vi "Swerve Wheel.vi"(7 "Wheel":T1(ring), 10 "Inputs":dbl[](array[numeric])) -> (1 "Speed":dbl, 2 "Motor Output":dbl)   [LabVIEW 2017]
uses:
  <vilib>/Rock Robotics/WPI/ThirdParty/Phoenix-LabVIEW/Motor Controller/Controls/CTRE_Phoenix_MotorControl_ControlMode.ctl
  <vilib>/Rock Robotics/Network Tables/NT Read Number.vi
  <vilib>/Rock Robotics/Network Tables/NT Write Number.vi
  <vilib>/Rock Robotics/Network Tables/NT Read Numeric Array.vi
  <vilib>/addons/control/pid/pid.llb/PID (DBL).vi
  <vilib>/addons/control/pid/NI_PID_pid.lvlib
panel:
  out "PID Values":cluster{"P":dbl, "I":dbl, "D":dbl}
  # "Swerve Wheel Control\nFRC Team 34"
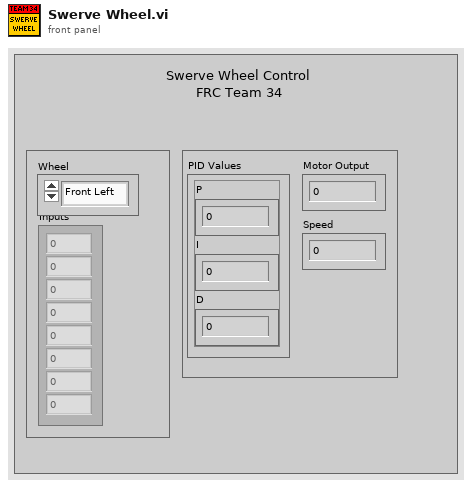
[diagram p1: front panel]
types:
  T1 = enum16{"Front Left", "Front Right", "Back Left", "Back Right"}
  T2 = enum16{"Z Axis", "Y", "X", "Rot. Point X", "Rot. Point Y", "Width/2", "Max", "Length/2"}
  T3 = typedef "CTRE_Phoenix_MotorControl_ControlMode.ctl" = u16
  T4 = enum16{"Z", "Y", "X", "Rot. Point X", "Rot. Point Y", "Width/2", "Max", "Length/2"}
  T5 = typedef "WPI_MotorControlDeviceRef.ctl" = cluster{"DeviceStatus":errorcluster, "Type":T6, "PWM":cluster{"PWM Channel":T7, "DeadBand":T8}, "CAN":cluster{"Device Number":u8, "SetOutput VI Ref":variant, "GetOutput VI Ref":variant, "Enable VI Ref":variant, "Disable VI Ref":variant, "Data":variant}, "Invert":bool, "DIO PWM":cluster{"PWM \"Enable\" Channel":T7, "DIOChannel":T9, "PWM Rate":dbl}}
  T6 = typedef "WPI_MotorControlType.ctl" = enum16{"PWM", "CAN", "DIO PWM"}
  T7 = typedef "FPGA_DIOPWMChannel.ctl" = enum8{"PWM 0", "PWM 1", "PWM 2", "PWM 3", "PWM 4", "PWM 5", "PWM 6", "PWM 7", "PWM 8", "PWM 9", "PWM MXP 0", "PWM MXP 1", "PWM MXP 2", "PWM MXP 3", "PWM MXP 4", "PWM MXP 5", "PWM MXP 6", "PWM MXP 7", "PWM MXP 8", "PWM MXP 9", "Invalid"}
  T8 = typedef "WPI_PWMDeadband.ctl" = cluster{"Name":string, "maxPositivePwm":i32, "minPositivePwm":i32, "centerPwm":i32, "maxNegativePwm":i32, "minNegativePwm":i32, "angularRange":u16}
  T9 = typedef "FPGA_DIOChannel.ctl" = enum8{"DIO 0", "DIO 1", "DIO 2", "DIO 3", "DIO 4", "DIO 5", "DIO 6", "DIO 7", "DIO 8", "DIO 9", "DIO MXP 0", "DIO MXP 1", "DIO MXP 2", "DIO MXP 3", "DIO MXP 4", "DIO MXP 5", "DIO MXP 6", "DIO MXP 7", "DIO MXP 8", "DIO MXP 9", "DIO MXP 10", "DIO MXP 11", "DIO MXP 12", "DIO MXP 13", "DIO MXP 14", "DIO MXP 15", "SPI Port CS1", "SPI Port CS2", "SPI Port CS3", "SPI Port MISO", "SPI Port MOSI", "Invalid"}
  T10 = typedef "WPI_EncoderDevRef.ctl" = cluster{"DevStatus":errorcluster, "EncoderIndex":T11, "CounterIndex":T12, "DistancePerCount":dbl, "Decoding Type":T13}
  T11 = typedef "FPGA_EncoderIdx.ctl" = enum8{"Enc 0", "Enc 1", "Enc 2", "Enc 3", "Enc 4", "Enc 5", "Enc 6", "Enc 7", "Invalid"}
  T12 = typedef "FPGA_CounterCtrSystemIndex.ctl" = enum8{"Ctr 0", "Ctr 1", "Ctr 2", "Ctr 3", "Ctr 4", "Ctr 5", "Ctr 6", "Ctr 7", "Invalid"}
  T13 = typedef "WPI_EncoderType.ctl" = enum16{"1x", "2x", "4x"}
  T14 = cluster{"Numeric":dbl, "Numeric":dbl, "Numeric":dbl}
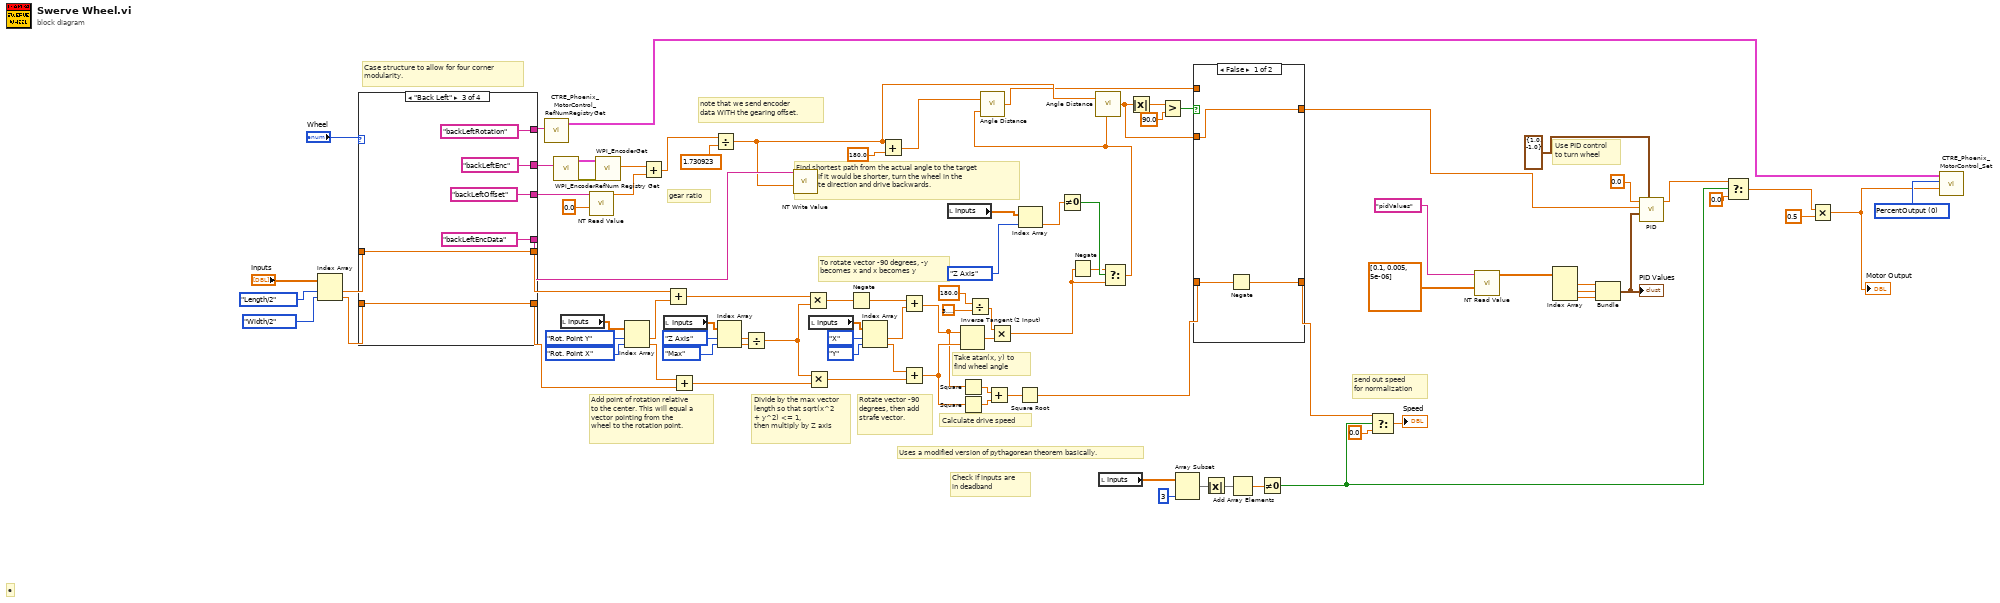
[diagram p0: block diagram]
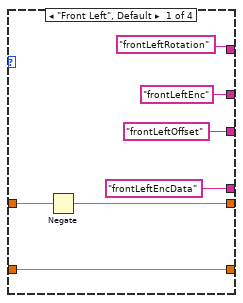
[diagram p3: hidden frame]
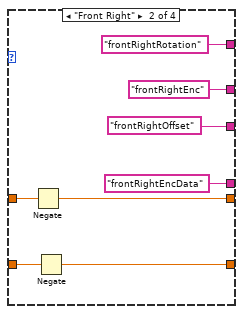
[diagram p4: hidden frame]
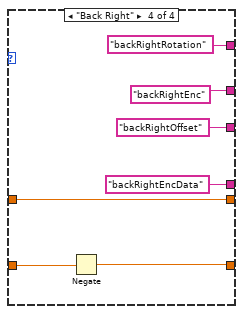
[diagram p5: hidden frame]
diagram:
  w31 = T3 0 items=["PercentOutput"=0, "Position"=1, "Velocity"=2, "Current"=3, "Follower"=5, "MotionProfile"=6, "MotionMagic"=7, "MotionMagicArc"=8, "MotionProfileArc"=10, "Disabled"=15] ("Control Mode")
  # "gear ratio"
  # "Uses a modified version of pythagorean theorem basically."
  # "e"
  # "note that we send encoder \ndata WITH the gearing offset."
  # "Case structure to allow for four corner\nmodularity."
  # "To rotate vector -90 degrees, -y becomes x and x becomes y"
  # "send out speed\nfor normalization"
  # "Use PID control\nto turn wheel"
  # "Find shortest path from the actual angle to the target angle. If it would be shorter, turn the wheel in the opposite direction and drive backwards."
  # "Divide by the max vector length so that sqrt(x^2 + y^2) <= 1,\nthen multiply by Z axis"
  # "Add point of rotation relative to the center. This will equal a vector pointing from the\nwheel to the rotation point."
  # "Check if inputs are\nin deadband"
  # "Take atan(x, y) to find wheel angle"
  # "Calculate drive speed"
  # "Rotate vector -90 degrees, then add strafe vector."
  n1 = Index Array(array="Inputs", index #1=T4."Length/2", index #2=T4."Width/2") -> (element #1=w87:dbl, element #2=w86:dbl)
  n2 = case shown="\"Back Left\"" "Wheel" {
    tunnel: w87 -> [w98 w106 w112 w119]
    tunnel: w86 -> [w96 w104 w111 w118]
    tunnel: [w97 w105 w112 w119] -> w56
    tunnel: [w96 w103 w111 w117] -> w55
    tunnel: ["frontLeftRotation" "frontRightRotation" "backLeftRotation" "backRightRotation"] -> w33
    tunnel: ["frontLeftEnc" ("refnum name") "frontRightEnc" ("refnum name") "backLeftEnc" ("refnum name") "backRightEnc" ("refnum name")] -> w68
    tunnel: ["frontLeftOffset" ("Name") "frontRightOffset" ("Name") "backLeftOffset" ("Name") "backRightOffset" ("Name")] -> w64
    tunnel: ["frontLeftEncData" ("Name") "frontRightEncData" ("Name") "backLeftEncData" ("Name") "backRightEncData" ("Name")] -> w36
    frame "Front Left", Default {
      n3 = Negate(x=w98) -> (-x=w97:dbl)
    }
    frame "Front Right" {
      n4 = Negate(x=w106) -> (-x=w105:dbl)
      n5 = Negate(x=w104) -> (-x=w103:dbl)
    }
    frame "Back Left" {
    }
    frame "Back Right" {
      n6 = Negate(x=w118) -> (-x=w117:dbl)
    }
  }
  n7 = call <vilib>:"CTRE_Phoenix_MotorControl_RefNumRegistryGet.vi"("refnum name"=w33) -> ("PhoenixMotorControlDevRef"=w32:T5)  [unwired: 9 in, 1 out]
  n8 = call <vilib>:"WPI_EncoderRefNum Registry Get.vi"("refnum name"=w68) -> ("error out"=w67:errorcluster, "EncoderDevRef"=w66:T10)  [unwired: 9 in]
  n9 = local read "Inputs"() -> (w61:dbl[])
  n10 = call-poly <vilib>:"NT Read Value.vi"("Default Value"=0.0, "Name"=w64) -> ("Numeric"=w59:dbl)  [unwired: 8 in, 1 out]
  n11 = call <vilib>:"WPI_EncoderGet.vi"("error in (no error)"=w67, "EncoderDevRef"=w66) -> ("Distance"=w60:dbl)  [unwired: 4 in, 5 out]
  n12 = Index Array(array=w61, index #1=T4."Rot. Point Y", index #2=T4."Rot. Point X") -> (element #1=w57:dbl, element #2=w58:dbl)
  n13 = Add(x=w60, y=w59) -> (x+y=w35:dbl)
  n14 = local read "Inputs"() -> (w69:dbl[])
  n15 = Add(x=w56, y=w57) -> (x+y=w54:dbl)
  n16 = Add(x=w58, y=w55) -> (x+y=w78:dbl)
  n17 = Divide(x=w35, y=1.730923) -> (x/y=w24:dbl)
  n18 = Index Array(array=w69, index #1=T2."Z Axis", index #2=T4."Max") -> (element #1=w38:dbl, element #2=w37:dbl)
  n19 = Divide(x=w38, y=w37) -> (x/y=w15:dbl)
  n20 = call-poly <vilib>:"NT Write Value.vi"("Numeric"=w24, "Name"=w36) -> ()  [unwired: 9 in, 1 out]
  n21 = Multiply(x=w54, y=w15) -> (x*y=w71:dbl)
  n22 = Multiply(x=w15, y=w78) -> (x*y=w74:dbl)
  n23 = local read "Inputs"() -> (w41:dbl[])
  n24 = Negate(x=w71) -> (-x=w70:dbl)
  n25 = Index Array(array=w41, index #1=T4."X", index #2=T4."Y") -> (element #1=w40:dbl, element #2=w39:dbl)
  n26 = Add(x=w24, y=180.0) -> (x+y=w23:dbl)
  n27 = Add(x=w70, y=w40) -> (x+y=w72:dbl)
  n28 = Add(x=w39, y=w74) -> (x+y=w73:dbl)
  n29 = local read "Inputs"() -> (w13:dbl[])
  n30 = Inverse Tangent (2 Input)(1:w73, 2:w72) -> (0:w85:dbl)
  n31 = Square(x=w72) -> (x^2=w75:dbl)
  n32 = Square(x=w73) -> (x^2=w84:dbl)
  n33 = Divide(x=180.0 ("y"), y=3.141592653589793) -> (x/y=w82:dbl)
  n34 = Add(x=w75, y=w84) -> (x+y=w83:dbl)
  n35 = Multiply(x=w82, y=w85) -> (x*y=w8:dbl)
  n36 = Square Root(x=w83) -> (sqrt(x)=w21:dbl)
  n37 = Index Array(array=w13, index=T2."Z Axis") -> (element=w11:dbl)
  n38 = Not Equal To 0?(x=w11) -> (x != 0?=w10:bool)
  n39 = Negate(x=w8) -> (-x=w9:dbl)
  n40 = local read "Inputs"() -> (w49:dbl[])
  n41 = Select(t=w9, s=w10, f=w8) -> (s? t:f=w14:dbl)
  n42 = call "Angle Distance.vi"("Target Angle"=w14, "Current Angle"=w23) -> ("Distance"=w22:dbl)
  n43 = call "Angle Distance.vi"("Target Angle"=w14, "Current Angle"=w24) -> ("Distance"=w18:dbl)
  n44 = Absolute Value(x=w18) -> (abs(x)=w17:dbl)
  n45 = Greater?(x=w17, y=90.0) -> (0:w19:bool)
  n46 = Array Subset(array=w49, length=3) -> (w51:dbl[])  [unwired: 1 in]
  n47 = case shown="False" w19 {
    tunnel: w21 -> [w121 w123]
    tunnel: w18 -> [w122 _]
    tunnel: w22 -> [_ w124]
    tunnel: [w120 w123] -> w20
    tunnel: [w122 w124] -> w1
    frame False {
      n48 = Negate(x=w121) -> (-x=w120:dbl)
    }
    frame True {
    }
  }
  n49 = Absolute Value(x=w51) -> (abs(x)=w50:dbl[])
  n50 = Add Array Elements(numeric array=w50) -> (sum=w52:dbl)
  n51 = Not Equal To 0?(x=w52) -> (x != 0?=w42:bool)
  n52 = Select(t=w20, s=w42, f=0.0) -> (s? t:f=→"Speed":dbl)
  n53 = call-poly <vilib>:"NT Read Value.vi"("Default Value"=dbl[] [0.1, 0.005, 5e-06], "Name"="pidValues") -> ("Numeric Array"=w6:dbl[])  [unwired: 8 in, 1 out]
  n54 = Index Array(array=w6) -> (element #1=w30:dbl, element #2=w29:dbl, element #3=w28:dbl)  [unwired: 3 in]
  n55 = Bundle("Numeric"=w30, "Numeric"=w29, "Numeric"=w28) -> (w26:T14)  [unwired: 1 in]
  "PID Values" <- w26
  n56 = call-poly <vilib>:"PID.vi"("output range"=cluster{"output high":dbl, "output low":dbl} {"output high"=1.0, "output low"=-1.0}, "PID gains"=w26, "process variable"=w1, "setpoint"=0.0) -> ("output"=w44:dbl)  [unwired: 6 in, 1 out]
  n57 = Select(t=w44, s=w42, f=0.0) -> (s? t:f=w4:dbl)
  n58 = Multiply(x=w4, y=0.5) -> (x*y=w2:dbl)
  "Motor Output" <- w2
  n59 = call <vilib>:"CTRE_Phoenix_MotorControl_Set.vi"("Output"=w2, "Control Mode"=w31, "PhoenixMotorControlDevRef"=w32) -> ()  [unwired: 7 in, 2 out]
